vi "PCert-Container-ShutdownActors.vi"(8 "error in (no error)":errorcluster, 11 "ERP-Container-UI in":refnum<class "PCert-Container-UI.lvclass">) -> (0 "error out":errorcluster, 3 "ERP-Container-UI out":refnum<class "PCert-Container-UI.lvclass">)   [LabVIEW 2013, in "PCert-Container-UI.lvclass"]
uses:
  PCert-Container-UI.lvclass
  PCert-Container-UI.lvclass/PCert-Container-UI.ctl
  ftw-dataflow/Actor/src/Connector/FTW-ActorConnector.lvclass
  ftw-dataflow/Core/src/Time/FTW-Time-Uptime.vi
  ftw-dataflow/Core/src/Database/FTW-SQLite-PrepareStatement.vi
  ftw-dataflow/Core/src/Database/FTW-SQLite-LibraryFilepath.vi
  ftw-dataflow/Core/src/Database/FTW-SQLite-LibraryReturnValue.vi
  ftw-dataflow/Core/src/Error/FTW-ERR-StatusOK.vi
  ftw-dataflow/Core/src/Error/FTW-ERR-ThrowImpossibleError.vi
  ftw-dataflow/Core/utils/CodeGen/SQLite-Fetch/FTW-SQLite-Fetch.xnode
  ftw-dataflow/Core/src/Database/FTW-SQLite-Connector.lvclass
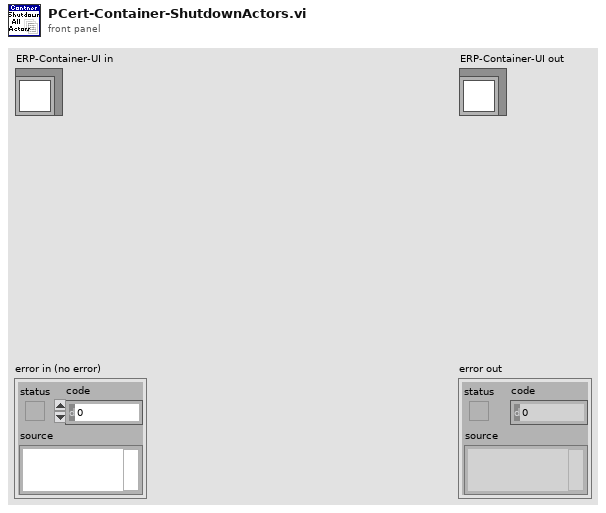
[diagram p1: front panel]
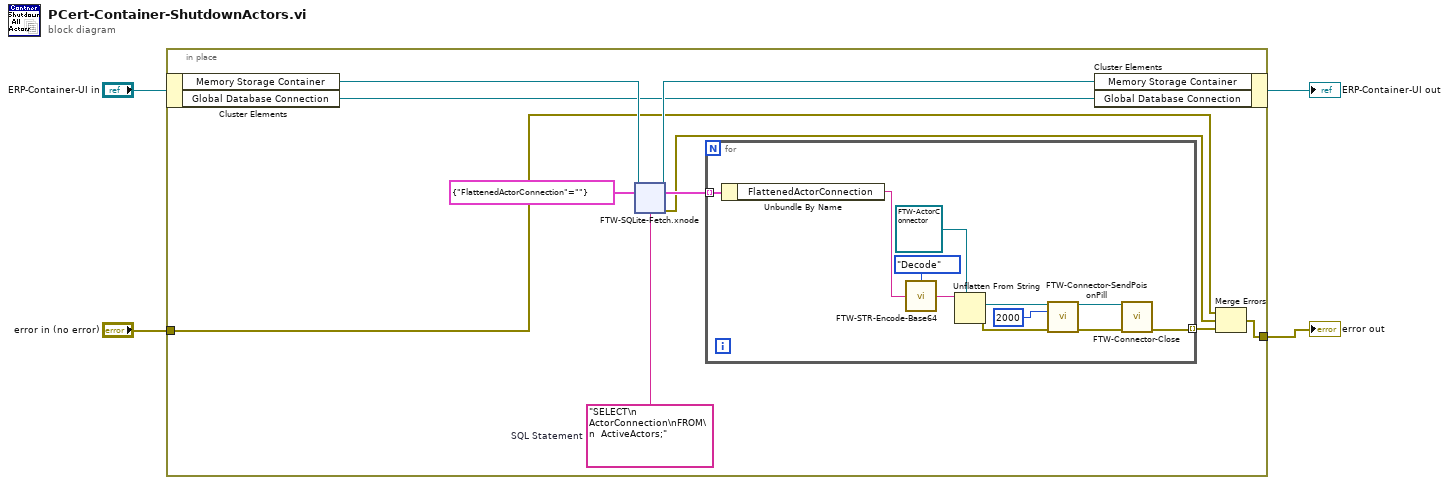
[diagram p0: block diagram]
diagram:
  n1 = in-place {
    in-place-border: "error in (no error)" -> [w5]
    in-place-border: [w8] -> w3
    w12 = "SELECT\n  ActorConnection\nFROM\n  ActiveActors;"  # SQL Statement
    n2 = in-place-cluster #1("ERP-Container-UI in") -> ("Memory Storage Container"=w13:refnum<class "FTW-SQLite-Connector.lvclass">, "Global Database Connection"=w6:refnum<class "FTW-ActorConnector.lvclass">)
    n3 = xnode "FTW-SQLite-Fetch.xnode"("SQLite Connector"=w13, "SQL Script"=w12, "Row Datatype"=cluster{"FlattenedActorConnection":string} {"FlattenedActorConnection"=""}) -> ("SQLite Connector out"=w10:refnum<class "FTW-SQLite-Connector.lvclass">, "Result Set"=w11:cluster{"FlattenedActorConnection":string}[], "error out"=w7:errorcluster)  [unwired: 1 in, 2 out]
    n4 = for {
      tunnel: w11 -> [w25] mode=indexing
      tunnel: [w15] -> w9 mode=indexing
      n5 = Unbundle By Name(w25) -> ("FlattenedActorConnection"=w23:string)
      n6 = call "FTW-STR-Encode-Base64.vi"("Input"=w23, "Direction"=enum16{"Encode", "Decode"}."Decode") -> ("Output"=w21:string)
      n7 = Unflatten From String(type=refnum<class "FTW-ActorConnector.lvclass"> refnum ("Featherweight Actor:FTW Actor Connector"), binary string=w21) -> (value=w19:refnum<class "FTW-ActorConnector.lvclass">, error out=w18:errorcluster)  [unwired: 3 in, 1 out]
      n8 = call-dynamic "FTW-Connector-SendPoisonPill.vi"("FTW Actor Connector"=w19, "Timeout"=2000, "error in"=w18) -> ("FTW Actor Connector out"=w16:refnum<class "FTW-ActorConnector.lvclass">, "error out"=w17:errorcluster)  [unwired: 8 in, 3 out]
      n9 = call-dynamic "FTW-Connector-Close.vi"("FTW Actor Connector"=w16, "error in"=w17) -> ("error out"=w15:errorcluster)  [unwired: 13 in]
    }
    n10 = in-place-cluster #1("Memory Storage Container"=w10, "Global Database Connection"=w6) -> (→"ERP-Container-UI out":refnum<class "PCert-Container-UI.lvclass">)
    n11 = Merge Errors(w5, w7, w9) -> (w8:errorcluster)
  }
  "error out" <- w3
